vi "Shutdown Queue.vi"(8 "Error in":errorcluster, 11 "Queue Data":T1) -> (0 "Error out":errorcluster)   [LabVIEW 2018, in "Queue Messaging.lvlib"]
uses:
  Queue Messaging.lvlib
  QMH Template/Type Defs/EventsAndQueues--cluster.ctl
  Type Defs/Queue Message--cluster.ctl
  Event Messaging/Type Defs/Event Message--cluster.ctl
  Event Messaging/Event Messaging.lvlib
  QMH/QMH CORE.lvlib
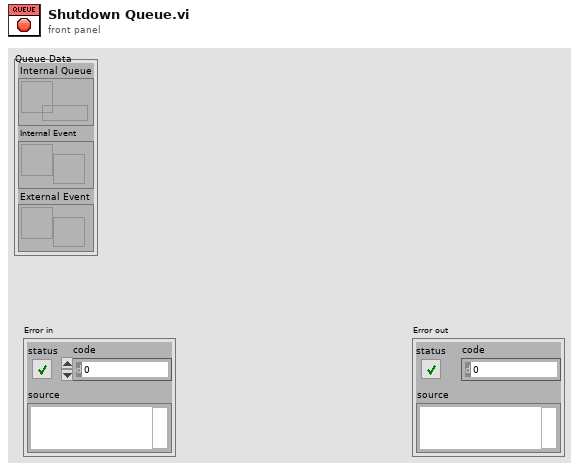
[diagram p1: front panel]
types:
  T1 = typedef "QMH CORE.lvlib/EventsAndQueues--cluster.ctl" = cluster{"Internal Queue":refnum<queue>, "Internal Event":refnum<user-event>, "External Event":refnum<user-event>}
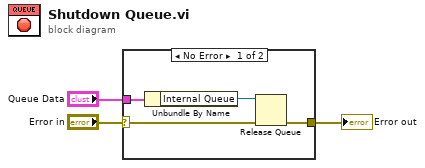
[diagram p0: block diagram]
diagram:
  n1 = case shown="No Error" "Error in" {
    selector: "Error in" -> [w5 w8]
    tunnel: "Queue Data" -> [w7 _]
    tunnel: [w4 w8] -> w1
    frame No Error {
      n2 = Unbundle By Name(w7) -> ("Internal Queue"=w6:refnum<queue>)
      n3 = Release Queue(queue=w6, error in (no error)=w5) -> (error out=w4:errorcluster)  [unwired: 1 in, 2 out]
    }
    frame Error {
    }
  }
  "Error out" <- w1
